vi "Rolling Image Average.vi"() -> ()   [LabVIEW 2023]
doc: "The Rolling Image Average example shows how to compute a rolling average while performing a ring acquisition. A queue is used to keep track of the image references used in the average. Once the queue becomes full, the oldest image reference is removed and released from the ring buffer.\n\nThis example requires NI Vision Development Module."
uses:
  <vilib>/vision/Image Controls.llb/IMAQ Image.ctl
  <vilib>/vision/driver/IMAQdx.llb/IMAQdx Acquisition Mode.ctl
  <vilib>/vision/driver/IMAQdx.llb/IMAQdx Buffer Number Mode.ctl
  <vilib>/vision/driver/NI_Vision_Acquisition_Software.lvlib
  <vilib>/vision/NI_Vision_Development_Module.lvlib
panel:
  in  "Number of Images to Average":i32=5
  out "Buffer Number":u32
  out "Rolling Average":T1(plugin-control)
  in  "Stop":bool
  in  "Camera Name":refnum<k21> caption="IMAQdx Session"
  # "Overview: Demonstrates how to compute a rolling average while doing a ring acquisition.\nRequirements:\n- Vision Acquisition Software\n- Vision Development Module\n- Camera configured with a Mono8 pixel format\nInstructions:\n1. Select the Camera Name\n2. Run the VI"
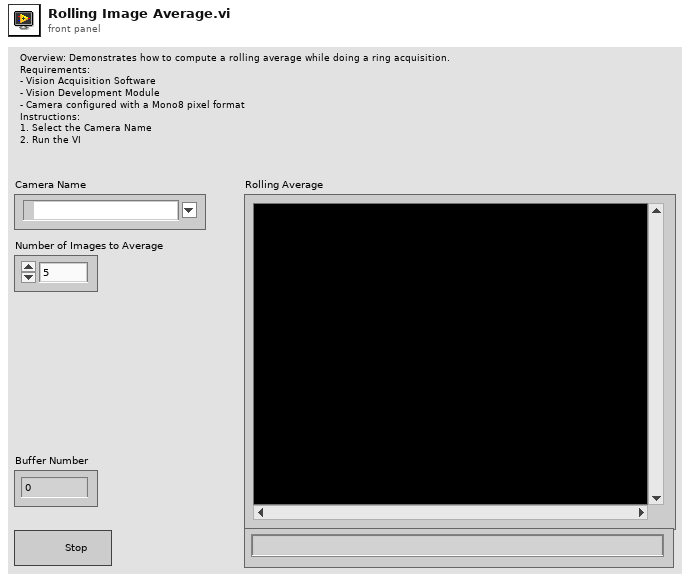
[diagram p1: front panel]
types:
  T1 = typedef "IMAQ Image.ctl" = refnum<image>
  T2 = typedef "NI_Vision_Acquisition_Software.lvlib/IMAQdx Acquisition Mode.ctl" = enum32{"One Shot", "Continuous"}
  T3 = typedef "NI_Vision_Acquisition_Software.lvlib/IMAQdx Buffer Number Mode.ctl" = enum32{"Next", "Last", "Buffer Number", "Every", "Last New"}
  T4 = typedef "Image Type" = u32
  T5 = typedef "IMAQdx.ctl" = refnum<k21>
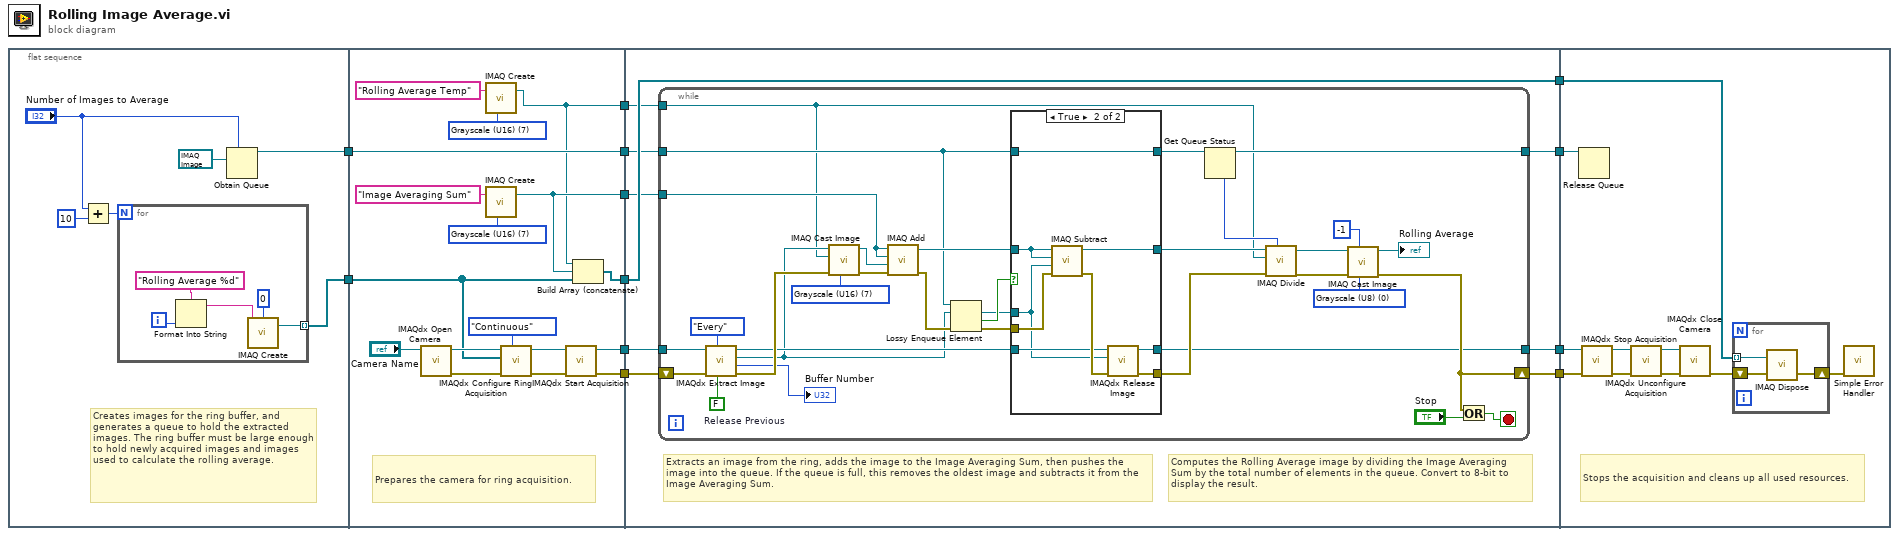
[diagram p0: block diagram]
diagram:
  n1 = flat-sequence {
    tunnel: [w15] -> w12
    tunnel: [w14] -> w11
    tunnel: w12 -> [w27]
    tunnel: w11 -> [w32]
    tunnel: [w34] -> w10
    tunnel: [w33] -> w9
    tunnel: [w32] -> w8
    tunnel: [w25] -> w7
    tunnel: [w26] -> w3
    tunnel: [w24] -> w1
    tunnel: w10 -> [w48]
    tunnel: w9 -> [w47]
    tunnel: w8 -> [w46]
    tunnel: w7 -> [w45]
    tunnel: [w44] -> w6
    tunnel: [w43] -> w5
    tunnel: [w42] -> w4
    tunnel: w3 -> [w49]
    tunnel: [w49] -> w2
    tunnel: w1 -> [w41]
    tunnel: w6 -> [w100]
    tunnel: w5 -> [w101]
    tunnel: w4 -> [w99]
    tunnel: w2 -> [w96]
    frame #0 {
      # "Creates images for the ring buffer, and generates a queue to hold the extracted images. The ring buffer must be large enough to hold newly acquired images and images used to calculate the rolling average."
      n2 = Add(x="Number of Images to Average", y=10) -> (x+y=w17:i32)
      n3 = for {
        N: w17 -> [_]
        tunnel: [w23] -> w15 mode=indexing
        i -> [w22]
        n4 = Format Into String(format string="Rolling Average %d" ("Image Name"), w22) -> (resulting string=w21:string)  [unwired: 2 in, 1 out]
        n5 = call "IMAQ Create"("Border Size"=0, "Image Name"=w21) -> ("New Image"=w23:T1)  [unwired: 2 in, 2 out]
      }
      n6 = Obtain Queue(max queue size (-1, unlimited)="Number of Images to Average", element data type=T1 refnum ("New Image")) -> (queue out=w14:refnum<queue>)  [unwired: 3 in, 2 out]
    }
    frame #1 {
      w29 = T4 7 items=["Grayscale (U8)", "Grayscale (I16)", "Grayscale (SGL)", "Complex (CSG)", "RGB (U32)", "HSL (U32)", "RGB (U64)", "Grayscale (U16)"] ("Image Type")
      w30 = T4 7 items=["Grayscale (U8)", "Grayscale (I16)", "Grayscale (SGL)", "Complex (CSG)", "RGB (U32)", "HSL (U32)", "RGB (U64)", "Grayscale (U16)"] ("Image Type")
      # "Prepares the camera for ring acquisition."
      n7 = call <vilib>:"IMAQdx Open Camera.vi"("Session In"="Camera Name") -> ("error out"=w39:errorcluster, "Session Out"=w38:T5)  [unwired: 2 in, 7 out]
      n8 = call "IMAQ Create"("Image Name"="Rolling Average Temp", "Image Type"=w29) -> ("New Image"=w24:T1)  [unwired: 3 in, 1 out]
      n9 = call "IMAQ Create"("Image Name"="Image Averaging Sum", "Image Type"=w30) -> ("New Image"=w25:T1)  [unwired: 3 in, 1 out]
      n10 = call <vilib>:"IMAQdx Configure Ring Acquisition.vi"("Mode"=IMAQdx_Acquisition_Mode."Continuous" ("Continuous?"), "error in"=w39, "Images"=w27, "Session In"=w38) -> ("error out"=w36:errorcluster, "Session Out"=w35:T5)  [unwired: 5 in, 1 out]
      n11 = call <vilib>:"IMAQdx Start Acquisition.vi"("error in"=w36, "Session In"=w35) -> ("error out"=w34:errorcluster, "Session Out"=w33:T5)  [unwired: 8 in]
      n12 = Build Array (concatenate)(w24, w25, w27) -> (w26:T1[])
    }
    frame #2 {
      # "Computes the Rolling Average image by dividing the Image Averaging Sum by the total number of elements in the queue. Convert to 8-bit to display the result."
      # "Extracts an image from the ring, adds the image to the Image Averaging Sum, then pushes the image into the queue. If the queue is full, this removes the oldest image and subtracts it from the Image Averaging Sum."
      n13 = while {
        tunnel: w47 -> [w80]
        tunnel: w46 -> [w70]
        shift-right: [w82] -> w43
        shift-left: w48 -> [w79]
        tunnel: [w60] -> w44
        tunnel: w45 -> [w59]
        tunnel: [w64] -> w42
        tunnel: w41 -> [w53]
        stop <- w65 stop-if-true
        w56 = T4 7 items=["Grayscale (U8)", "Grayscale (I16)", "Grayscale (SGL)", "Complex (CSG)", "RGB (U32)", "HSL (U32)", "RGB (U64)", "Grayscale (U16)"] ("Image Type")
        w62 = T4 0 items=["Grayscale (U8)", "Grayscale (I16)", "Grayscale (SGL)", "Complex (CSG)", "RGB (U32)", "HSL (U32)", "RGB (U64)", "Grayscale (U16)"] ("Image Type")
        w78 = FALSE  # Release Previous
        n14 = call <vilib>:"IMAQdx Extract Image.vi"("Release Previous (true)"=w78, "Buffer Number Mode (Next)"=IMAQdx_Buffer_Number_Mode."Every", "error in"=w79, "Session In"=w80) -> ("error out"=w81:errorcluster, "Buffer Number Out"=→"Buffer Number":u32, "Image Out"=w57:T1, "Session Out"=w73:T5)  [unwired: 4 in]
        n15 = call "IMAQ Cast Image"("Image Type"=w56, "error in (no error)"=w81, "Image Dst"=w53, "Image Src"=w57) -> ("error out"=w58:errorcluster, "Image Dst Out"=w55:T1)  [unwired: 6 in]
        n16 = call "IMAQ Add"("Image Src A"=w59, "Image Dst"=w59, "Image Src B"=w55, "error in (no error)"=w58) -> ("Image Dst Out"=w72:T1, "error out"=w76:errorcluster)  [unwired: 3 in]
        n17 = Lossy Enqueue Element(queue=w70, element=w57, error in (no error)=w76) -> (overflow element=w74:T1, overflow?=w75:bool, error out=w71:errorcluster)  [unwired: 1 out]
        n18 = case shown="True" w75 {
          tunnel: w74 -> [_ w91]
          tunnel: w73 -> [w86 w93]
          tunnel: w72 -> [w84 w94]
          tunnel: w71 -> [w85 w92]
          tunnel: [w85 w90] -> w67
          tunnel: [w86 w89] -> w60
          tunnel: [w84 w88] -> w54
          tunnel: [w83 w87] -> w69
          tunnel: w70 -> [w83 w87]
          frame False {
          }
          frame True {
            n19 = call "IMAQ Subtract"("Image Src A"=w94, "Image Dst"=w94, "Image Src B"=w91, "error in (no error)"=w92) -> ("Image Dst Out"=w88:T1, "error out"=w95:errorcluster)  [unwired: 3 in]
            n20 = call <vilib>:"IMAQdx Release Image.vi"("error in"=w95, "Image"=w91, "Session In"=w93) -> ("error out"=w90:errorcluster, "Session Out"=w89:T5)  [unwired: 7 in]
          }
        }
        n21 = Get Queue Status(queue=w69) -> (queue out=w64:refnum<queue>, # elements in queue=w68:i32)  [unwired: 2 in, 6 out]
        n22 = call "IMAQ Divide"("Image Src A"=w54, "Constant"=w68, "Image Dst"=w53, "error in (no error)"=w67) -> ("Image Dst Out"=w52:T1, "error out"=w63:errorcluster)  [unwired: 3 in]
        n23 = call "IMAQ Cast Image"("Image Type"=w62, "# Shifts"=-1, "error in (no error)"=w63, "Image Src"=w52) -> ("error out"=w82:errorcluster, "Image Dst Out"=→"Rolling Average":T1)  [unwired: 6 in]
        n24 = Or(x=w82, y="Stop") -> (x .or. y?=w65:bool)
      }
    }
    frame #3 {
      # "Stops the acquisition and cleans up all used resources."
      n25 = Release Queue(queue=w99) -> ()  [unwired: 2 in, 3 out]
      n26 = call <vilib>:"IMAQdx Stop Acquisition.vi"("error in"=w101, "Session In"=w100) -> ("error out"=w105:errorcluster, "Session Out"=w104:T5)  [unwired: 8 out]
      n27 = call <vilib>:"IMAQdx Unconfigure Acquisition.vi"("error in"=w105, "Session In"=w104) -> ("error out"=w102:errorcluster, "Session Out"=w103:T5)  [unwired: 8 out]
      n28 = call <vilib>:"IMAQdx Close Camera.vi"("error in"=w102, "Session In"=w103) -> ("error out"=w98:errorcluster)  [unwired: 9 out]
      n29 = for {
        shift-right: [w107] -> w97
        shift-left: w98 -> [w108]
        tunnel: w96 -> [w106] mode=indexing
        n30 = call "IMAQ Dispose"("Image"=w106, "error in (no error)"=w108) -> ("error out"=w107:errorcluster)  [unwired: 4 in]
      }
      n31 = call <vilib>:"Simple Error Handler.vi"("error in (no error)"=w97) -> ()  [unwired: 4 in, 5 out]
    }
  }
